vi "max_min_array_elmnt.vi"() -> ()   [LabVIEW 2026]
panel:
  in  "Array":dbl[](array[numeric])
  out "min_val_index":dbl
  out "min_val":dbl
  out "max_val_index":dbl
  out "max_val":dbl
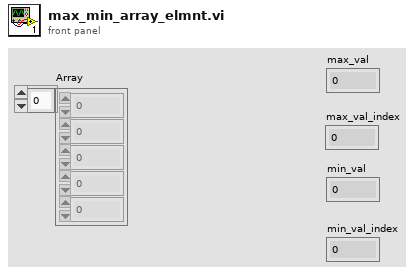
[diagram p1: front panel]
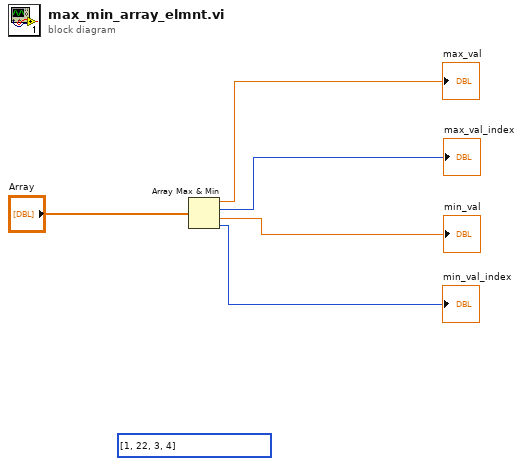
[diagram p0: block diagram]
diagram:
  (unwired) i32[] [1, 22, 3, 4]
  n1 = Array Max & Min(array="Array") -> (max value=→"max_val":dbl, max index (indices)=→"max_val_index":i32, min value=→"min_val":dbl, min index (indices)=→"min_val_index":i32)
